vi "Pause.vi"(7 "[x]":T1, 8 "error in (no error)":errorcluster, 11 "Serial Port in":refnum<visa-resource-name>) -> (0 "error out":errorcluster, 3 "Serial Port out":refnum<visa-resource-name>)   [LabVIEW 2016, in "Chemyx_Syringe_Pump_driver.lvlib"]
doc: "Pauses the current operation of the pump."
uses:
  Chemyx_Syringe_Pump_driver.lvlib
  _private/Control/Control Mode.ctl
panel:
  # "Pauses the current operation of the pump."
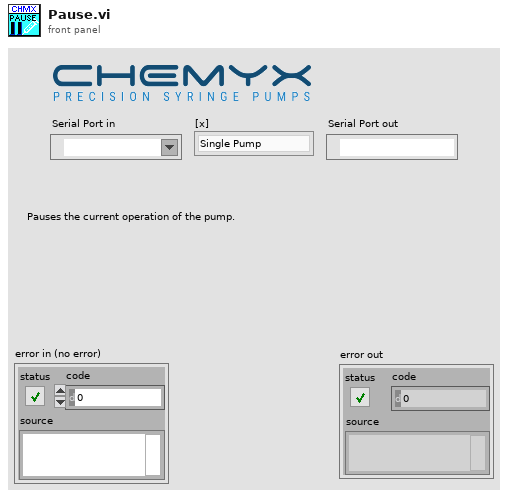
[diagram p1: front panel]
types:
  T1 = typedef "Chemyx_Syringe_Pump_driver.lvlib/Control Mode.ctl" = enum16{"Single Pump", "Pump Chanel 1", "Pump Channel 2", "Cycle Mode"}
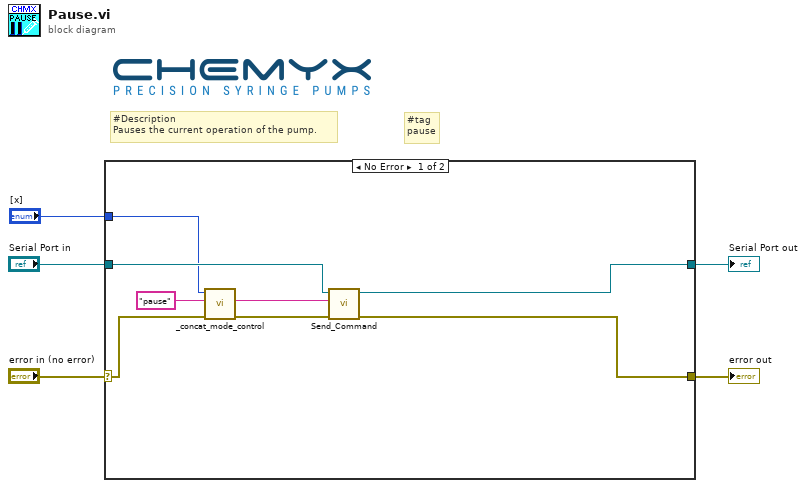
[diagram p0: block diagram]
diagram:
  # "#tag\npause"
  # "#Description\nPauses the current operation of the pump."
  n1 = case shown="No Error" "error in (no error)" {
    selector: "error in (no error)" -> [w11 w14]
    tunnel: "Serial Port in" -> [w12 w13]
    tunnel: [w10 w14] -> w3
    tunnel: [w9 w13] -> w2
    tunnel: "[x]" -> [w6 _]
    frame No Error {
      n2 = call "_concat_mode_control.vi"("write buffer"="pause", "[x]"=w6) -> ("write buffer out"=w7:string)  [unwired: 9 in]
      n3 = call "Send_Command.vi"("error in (no error)"=w11, "write buffer"=w7, "Serial Port in"=w12) -> ("error out"=w10:errorcluster, "VISA Refnum out"=w9:refnum<visa-resource-name>)  [unwired: 6 in, 1 out]
    }
    frame Error {
    }
  }
  "error out" <- w3
  "Serial Port out" <- w2
